vi "Store Operator.vi"(9 "Command":T1=enum."Initialize", 11 "String":string) -> (3 "Array":string[](array[string]))   [LabVIEW 2019]
uses:
  control/command control.ctl
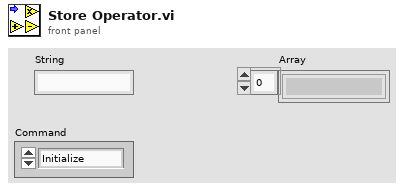
[diagram p1: front panel]
types:
  T1 = typedef "command control.ctl" = enum16{"Multiply", "Divide", "Initialize", "Minus", "Equal", "Add", "Decimal Point", "Number"}
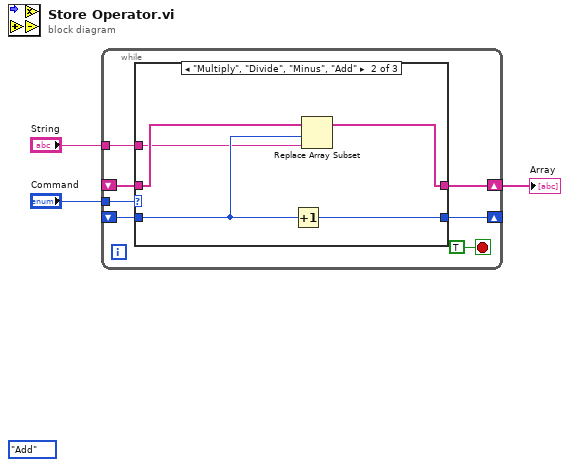
[diagram p0: block diagram]
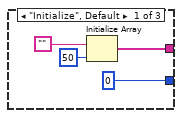
[diagram p2: hidden frame]
diagram:
  (unwired) command_control."Add" ("Command")
  n1 = while {
    shift-right: [w4] -> w2
    shift-left: _ -> [w9]
    tunnel: "Command" -> [w8]
    shift-right: [w7] -> _
    shift-left: _ -> [w6]
    tunnel: "String" -> [w5]
    stop <- TRUE stop-if-true
    n2 = case shown="\"Multiply\", \"Divide\", \"Minus\", \"Add\"" w8 {
      tunnel: [w11 w15 w21] -> w4
      tunnel: w9 -> [_ w17 w21]
      tunnel: [0 ("dimension size") w19 w20] -> w7
      tunnel: w6 -> [_ w18 w20]
      tunnel: w5 -> [_ w16 _]
      frame "Initialize", Default {
        n3 = Initialize Array("", 50 ("dimension size")) -> (w11:string[])
      }
      frame "Multiply", "Divide", "Minus", "Add" {
        n4 = Increment(x=w18) -> (x+1=w19:i32)
        n5 = Replace Array Subset(array=w17, new element=w16, index=w18) -> (w15:string[])
      }
      frame "Equal" {
      }
    }
  }
  "Array" <- w2
